vi "virtual XYZ rotator.vi"(0 "vertical (cw is pos)":dbl=nan, 1 "current pos X":dbl, 2 "current pos Y":dbl, 3 "current pos Z":dbl, 5 "horizontal (cw is pos)":dbl=nan, 12 "virtual X relative":dbl, 13 "virtual Y relative":dbl, 14 "virtual Z relative":dbl) -> (6 "new pos X":dbl=nan, 8 "new pos Y":dbl=nan, 10 "new pos Z":dbl=nan)   [LabVIEW 2012]
uses:
  <vilib>/Analysis/coordinate.llb/Euler Rotation Order.ctl
  <vilib>/Analysis/coordinate.llb/3D Cartesian Coordinate Rotation (Euler) (Scalar).vi
  GFG/GFGnumericGet.vi
  <vilib>/Analysis/NI_AALPro.lvlib
  GFG/GFG library.lvlib
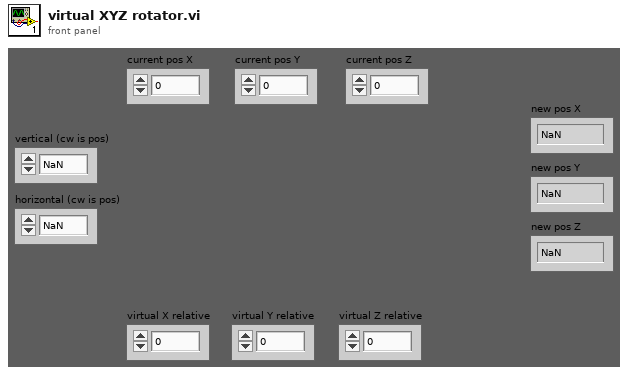
[diagram p1: front panel]
types:
  T1 = cluster{"phi":dbl, "vertical (cw is pos)":dbl, "horizontal (cw is pos)":dbl}
  T2 = typedef "NI_AALPro.lvlib/Euler Rotation Order.ctl" = u16
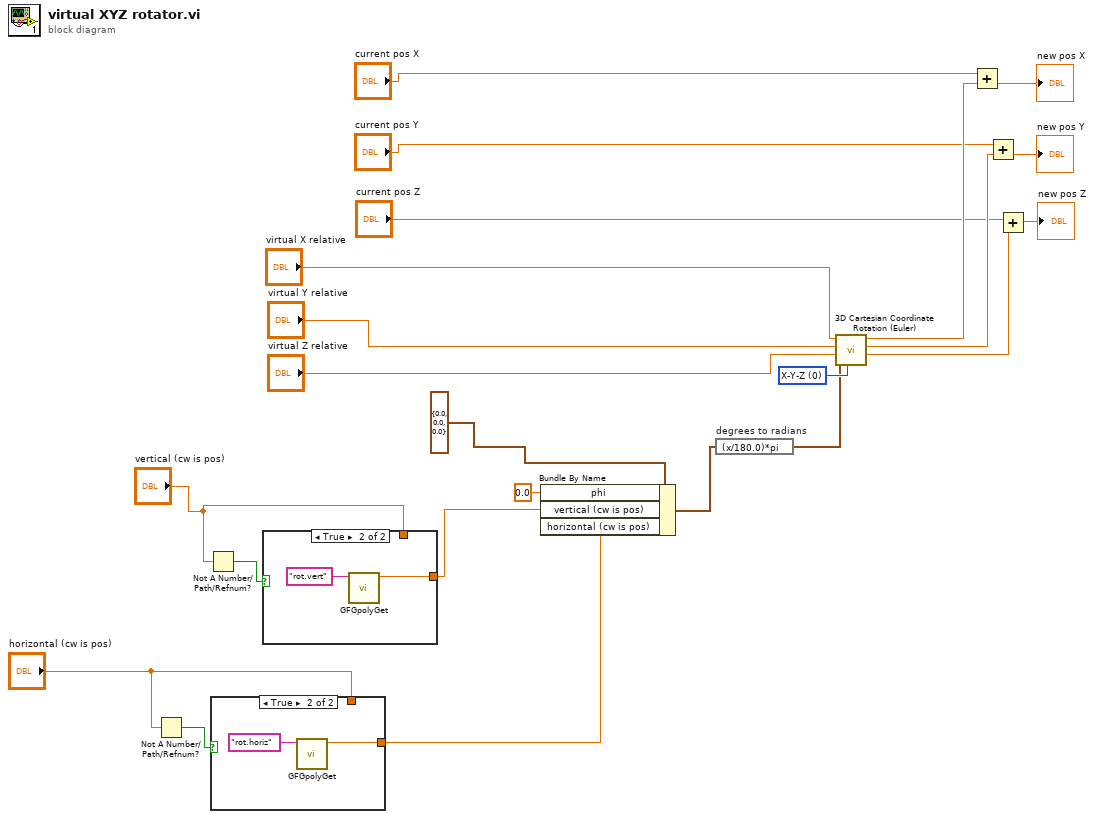
[diagram p0: block diagram]
diagram:
  w23 = T2 0 items=["X-Y-Z", "X-Z-Y", "Y-X-Z", "Y-Z-X", "Z-X-Y", "Z-Y-X", "X-Y-X", "X-Z-X", "Y-X-Y", "Y-Z-Y", "Z-X-Z", "Z-Y-Z"] ("rotation order")
  n1 = Not A Number/Path/Refnum?(number/path/refnum="horizontal (cw is pos)") -> (NaN/Path/Refnum?=w6:bool)
  n2 = Not A Number/Path/Refnum?(number/path/refnum="vertical (cw is pos)") -> (NaN/Path/Refnum?=w3:bool)
  n3 = case shown="True" w6 {
    tunnel: [w24 w25] -> w4
    tunnel: "horizontal (cw is pos)" -> [w24 _]
    frame False {
    }
    frame True {
      n4 = call-poly "GFGpolyGet.vi"("Variable Name in"="rot.horiz") -> ("Numeric"=w25:dbl)  [unwired: 9 in, 1 out]
    }
  }
  n5 = case shown="True" w3 {
    tunnel: [w27 w28] -> w1
    tunnel: "vertical (cw is pos)" -> [w27 _]
    frame False {
    }
    frame True {
      n6 = call-poly "GFGpolyGet.vi"("Variable Name in"="rot.vert") -> ("Numeric"=w28:dbl)  [unwired: 9 in, 1 out]
    }
  }
  n7 = Bundle By Name(cluster=T1 {"phi"=0.0, "vertical (cw is pos)"=0.0, "horizontal (cw is pos)"=0.0} ("Euler Angles (in degrees)"), "phi"=0.0, "vertical (cw is pos)"=w1, "horizontal (cw is pos)"=w4) -> (w21:T1)
  n8 = expression code="(x/180.0)*pi" "degrees to radians"(w21) -> (w20:T1)
  n9 = call-poly <vilib>:"3D Cartesian Coordinate Rotation (Euler).vi"("rotation order"=w23, "Euler Angles"=w20, "z"="virtual Z relative", "y"="virtual Y relative", "x"="virtual X relative") -> ("z out"=w18:dbl, "y out"=w17:dbl, "x out"=w16:dbl)  [unwired: 3 in, 1 out]
  n10 = Add(x="current pos X", y=w16) -> (x+y=→"new pos X":dbl)
  n11 = Add(x="current pos Y", y=w17) -> (x+y=→"new pos Y":dbl)
  n12 = Add(x="current pos Z", y=w18) -> (x+y=→"new pos Z":dbl)
